vi "CR-衬丝检测参数读取.vi"(7 "error in (no error)":errorcluster caption="错误输入（无错误）", 10 "基路径":path) -> (0 "error out":errorcluster caption="错误输出", 1 "CR- 衬丝检测参数":T6={"Settings (Clamp (Rake) 1)"={"Contrast"=154, "Filter width"=4, "Steepness"=2, "Subsampling Ratio"=5, "Show Search Area"=TRUE, "Show Search Lines"=TRUE, "Show Edges Found"=TRUE, "Show Result"=TRUE}, "Options (Find Straight Edge 1)"={"Search Direction"=0, "Edge Options"={"Edge Polarity"=0, "Kernel Size"=3, "Width"=1, "Minimum Edge Strength"=65.0, "Interpolation Type"=enum."Bilinear Fixed", "Data Processing Method"=enum."Average"}, "Show Search Area"=TRUE, "Show Search Lines"=TRUE, "Show Edges Found"=TRUE, "Show Result"=TRUE, "Search Area Color"=65280, "Search Lines Color"=255, "Edge Locations Color"=16776960, "Result Color"=16711680, "Overlay Group Name"=""}, "相对距离设定"={"上限"=0.0, "下限"=0.0}, "衬丝直径设定"={"上限"=0.0, "下限"=0.0}, "保护套直径设定"={"上限"=0.0, "下限"=0.0}, "Edge Options (Edge Detector 1)"={"Edge Polarity"=0, "Kernel Size"=3, "Width"=3, "Minimum Edge Strength"=10.0, "Interpolation Type"=enum."Bilinear Fixed", "Data Processing Method"=enum."Average"}, "保护套标准位置"={"Start X"=0, "Start Y"=0, "End X"=0, "End Y"=0}} {"保护套标准位置"."Start X" scale=0.0..1024.0; "保护套标准位置"."End X" scale=0.0..1024.0; "Edge Options (Edge Detector 1)"."Edge Polarity" items=["All Edges", "Rising Edges", "Falling Edges"]; "Options (Find Straight Edge 1)"."Search Direction" items=["Left to Right", "Right to Left", "Top to Bottom", "Bottom to Top"]; "Options (Find Straight Edge 1)"."Edge Options"."Edge Polarity" items=["All Edges", "Rising Edges", "Falling Edges"]; "Options (Find Straight Edge 1)"."Edge Options"."Minimum Edge Strength" format="%.2f"; "Options (Find Straight Edge 1)"."Edge Options"."Width" step=2; "Options (Find Straight Edge 1)"."Edge Options"."Kernel Size" step=2}, 2 "衬丝检测基础参数":T7={"IsNorImage"=TRUE, "Exposure Values"=100289, "ImagePath"=path "C:/Users/hedongpo/Desktop/514-hdp/Alignment Assemble System/Test Picture/B/3.bmp"} caption="参数界面" {"Exposure Values" scale=0.0..200000.0}, 3 "CR- 衬丝检测ROI参数":T3 {"Line 2"."Start X" scale=0.0..1024.0; "Line 2"."End X" scale=0.0..1024.0; "clamp Rectangle"."Rotation" min=-90.0 max=90.0 step=1.0 format="%.2f"; "clamp Rectangle"."Left" scale=0.0..1024.0; "clamp Rectangle"."Right" scale=0.0..1024.0; "Line 1"."Start X" scale=0.0..1024.0; "Line 1"."End X" scale=0.0..1024.0; "find straight edge Rectangle"."Rotation" min=-90.0 max=90.0 step=1.0 format="%.2f"; "find straight edge Rectangle"."Left" scale=0.0..1024.0; "find straight edge Rectangle"."Right" scale=0.0..1024.0})   [LabVIEW 2017]
uses:
  <vilib>/vision/Measure.llb/Edge Options.ctl
  <vilib>/vision/Measure.llb/Edge Polarity.ctl
  <vilib>/Utility/xml.llb/Read From XML File(string).vi
  Global System.vi
panel:
  # "UI电源线反面标签1基础参数"
  # "D:\\Inspect System\\Source Code\\Template Program\\BlackTemplete"
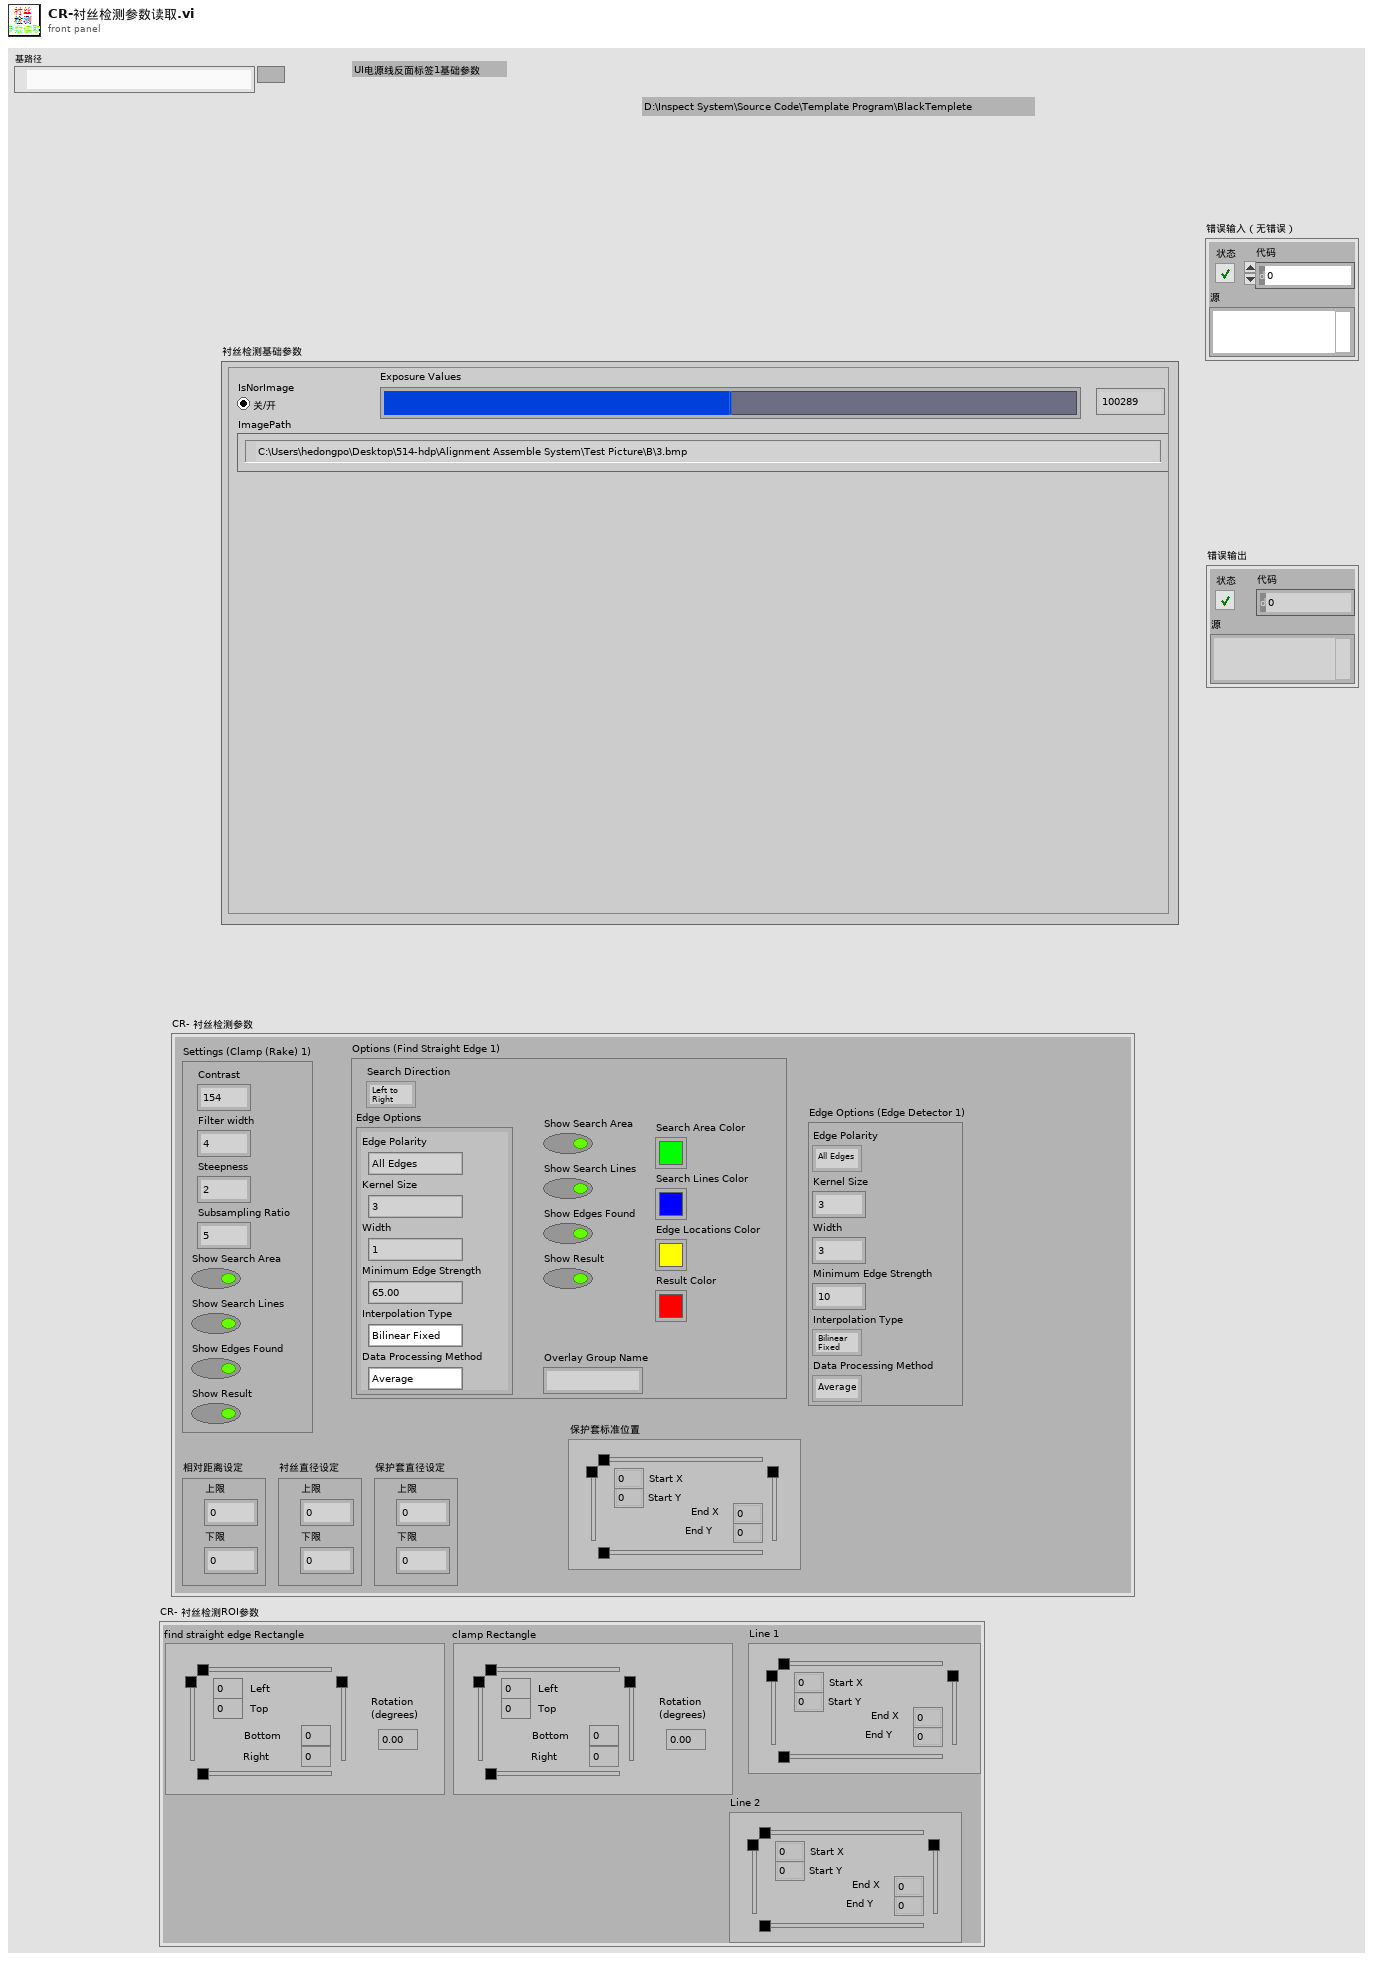
[diagram p1: front panel]
types:
  T1 = typedef "IMAQ Rectangle" = cluster{"Left":i32, "Top":i32, "Right":i32, "Bottom":i32, "Rotation":dbl}
  T2 = typedef "IMAQ Line" = cluster{"Start X":i32, "Start Y":i32, "End X":i32, "End Y":i32}
  T3 = cluster{"find straight edge Rectangle":T1, "Line 1":T2, "clamp Rectangle ":T1, "Line 2":T2}
  T4 = typedef "Edge Options.ctl" = cluster{"Edge Polarity":T5, "Kernel Size":u32, "Width":u32, "Minimum Edge Strength":sgl, "Interpolation Type":enum32{"Zero Order", "Bilinear", "Quadratic", "Cubic", "Bilinear Fixed"}, "Data Processing Method":enum32{"Average", "Median"}}
  T5 = typedef "Edge Polarity.ctl" = u32
  T6 = cluster{"Settings (Clamp (Rake) 1)":cluster{"Contrast":i32, "Filter width":i32, "Steepness":i32, "Subsampling Ratio":u32, "Show Search Area":bool, "Show Search Lines":bool, "Show Edges Found":bool, "Show Result":bool}, "Options (Find Straight Edge 1)":cluster{"Search Direction":u32, "Edge Options":T4, "Show Search Area":bool, "Show Search Lines":bool, "Show Edges Found":bool, "Show Result":bool, "Search Area Color":u32, "Search Lines Color":u32, "Edge Locations Color":u32, "Result Color":u32, "Overlay Group Name":string}, "相对距离设定":cluster{"上限":dbl, "下限":dbl}, "衬丝直径设定":cluster{"上限":dbl, "下限":dbl}, "保护套直径设定":cluster{"上限":dbl, "下限":dbl}, "Edge Options (Edge Detector 1)":cluster{"Edge Polarity":u32, "Kernel Size":u32, "Width":u32, "Minimum Edge Strength":sgl, "Interpolation Type":enum32{"Zero Order", "Bilinear", "Quadratic", "Cubic", "Bilinear Fixed"}, "Data Processing Method":enum32{"Average", "Median"}}, "保护套标准位置":T2}
  T7 = cluster{"IsNorImage":bool, "Exposure Values":u32, "ImagePath":path}
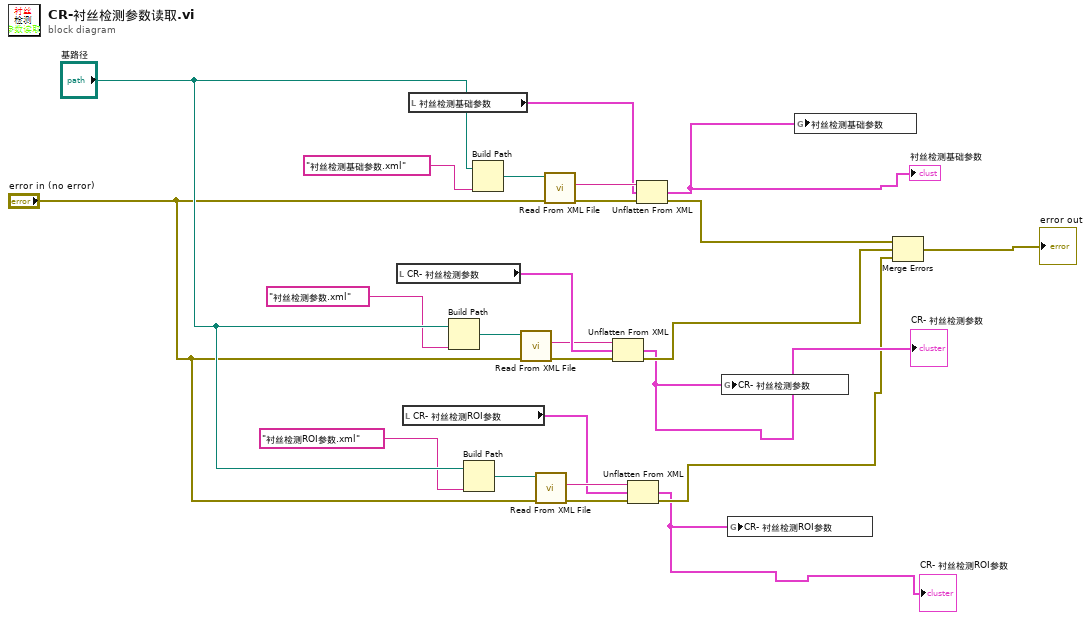
[diagram p0: block diagram]
diagram:
  n1 = local read "CR- 衬丝检测参数"() -> (w13:T6)
  n2 = local read "CR- 衬丝检测ROI参数"() -> (w3:T3)
  n3 = local read "衬丝检测基础参数"() -> (w22:T7)
  n4 = Build Path(base path="基路径", name or relative path="衬丝检测参数.xml" ("名称或相对路径")) -> (appended path=w11:path)
  n5 = Build Path(base path="基路径", name or relative path="衬丝检测ROI参数.xml" ("名称或相对路径")) -> (appended path=w5:path)
  n6 = Build Path(base path="基路径", name or relative path="衬丝检测基础参数.xml" ("名称或相对路径")) -> (appended path=w24:path)
  n7 = call-poly <vilib>:"Read From XML File.vi"("error in (no error)"="error in (no error)", "XML File Path"=w11) -> ("error out"=w10:errorcluster, "XML Elements"=w12:string)  [unwired: 7 in, 1 out]
  n8 = call-poly <vilib>:"Read From XML File.vi"("error in (no error)"="error in (no error)", "XML File Path"=w5) -> ("error out"=w6:errorcluster, "XML Elements"=w4:string)  [unwired: 7 in, 1 out]
  n9 = call-poly <vilib>:"Read From XML File.vi"("error in (no error)"="error in (no error)", "XML File Path"=w24) -> ("error out"=w21:errorcluster, "XML Elements"=w23:string)  [unwired: 7 in, 1 out]
  n10 = Unflatten From XML(xml string=w12, type=w13, error in (no error)=w10) -> (value=w8:T6, error out=w14:errorcluster)
  "CR- 衬丝检测参数" <- w8
  n11 = Unflatten From XML(xml string=w4, type=w3, error in (no error)=w6) -> (value=w1:T3, error out=w2:errorcluster)
  "CR- 衬丝检测ROI参数" <- w1
  n12 = Unflatten From XML(xml string=w23, type=w22, error in (no error)=w21) -> (value=w18:T7, error out=w20:errorcluster)
  "衬丝检测基础参数" <- w18
  n13 = global write "Global System.vi" "CR- 衬丝检测参数"(w8) -> ()
  n14 = global write "Global System.vi" "CR- 衬丝检测ROI参数"(w1) -> ()
  n15 = global write "Global System.vi" "衬丝检测基础参数"(w18) -> ()
  n16 = Merge Errors(w20, w14, w2) -> (→"error out":errorcluster)
